vi "Publish Trace.vi"(8 "error in (no error)":errorcluster, 10 "Trace":refnum<class "Trace.lvclass">, 11 "Trace Controller in":refnum<class "Trace Controller.lvclass">) -> (0 "error out":errorcluster, 3 "Trace Controller out":refnum<class "Trace Controller.lvclass">)   [LabVIEW 2014, in "Robot Actor Framework.lvlib" / "Trace.lvlib" / "Trace Controller.lvclass"]
uses:
  Trace Controller.lvclass
  Trace Class/Trace.lvclass
  Trace Controller.lvclass/Trace Controller.ctl
  Trace Listener Messages/Published Trace Msg/Published Trace Msg.lvclass/Published Trace Msg.ctl
  <vilib>/ActorFramework/Message Enqueuer/Message Enqueuer.lvclass/Message Enqueuer.ctl
  <vilib>/ActorFramework/Message Enqueuer/Enqueue.vi
  <vilib>/ActorFramework/Message Priority Queue/Priority Enqueue.vi
  Trace Listener Messages/Published Trace Msg/Published Trace Msg.lvclass
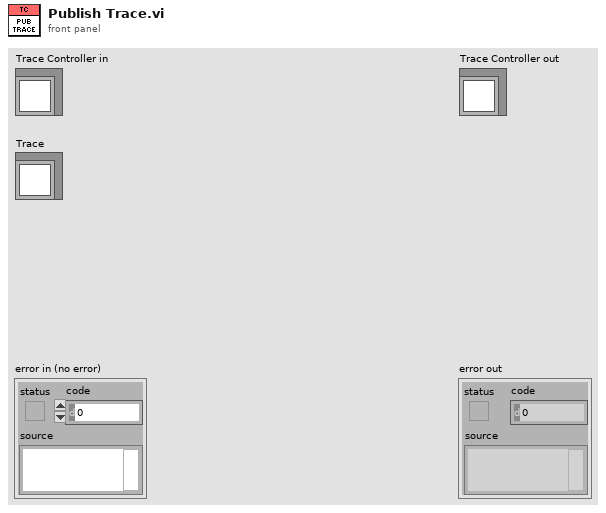
[diagram p1: front panel]
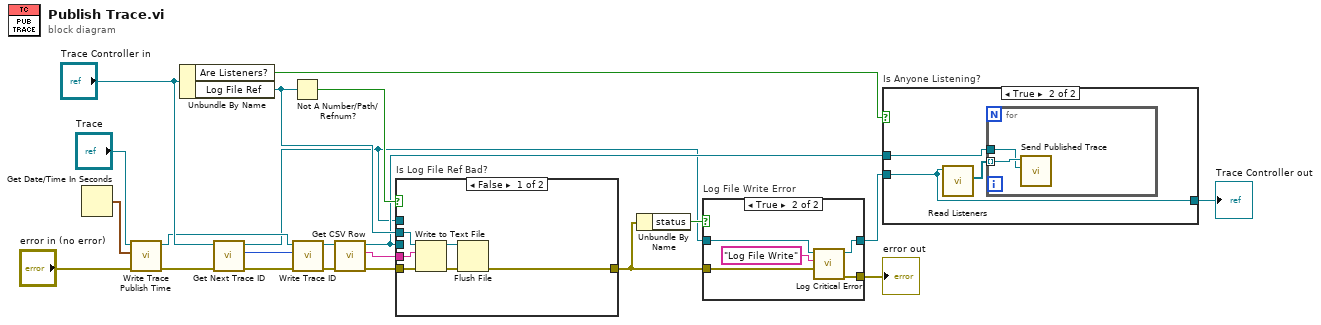
[diagram p0: block diagram]
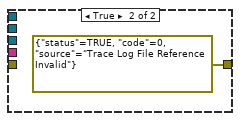
[diagram p2: hidden frame]
diagram:
  n1 = Get Date/Time In Seconds() -> (seconds since 1Jan1904=w19:timestamp)
  n2 = call-dynamic "Write Trace Publish Time.vi"("error in (no error)"="error in (no error)", "Trace Time"=w19, "Trace in"="Trace") -> ("error out"=w3:errorcluster, "Trace out"=w9:refnum<class "Trace.lvclass">)  [unwired: 7 in]
  n3 = Unbundle By Name("Trace Controller in") -> ("Are Listeners?"=w21:bool, "Log File Ref"=w12:refnum<file>)
  n4 = call-dynamic "Get Next Trace ID.vi"("error in (no error)"=w3, "Trace Controller in"="Trace Controller in") -> ("error out"=w2:errorcluster, "Next Trace ID"=w7:u64, "Trace Controller out"=w5:refnum<class "Trace Controller.lvclass">)  [unwired: 7 in]
  n5 = Not A Number/Path/Refnum?(number/path/refnum=w12) -> (NaN/Path/Refnum?=w11:bool)
  n6 = call-dynamic "Write Trace ID.vi"("error in (no error)"=w2, "Trace ID"=w7, "Trace in"=w9) -> ("error out"=w1:errorcluster, "Trace out"=w8:refnum<class "Trace.lvclass">)  [unwired: 7 in]
  n7 = call-dynamic "Get CSV Row.vi"("error in (no error)"=w1, "Trace in"=w8) -> ("error out"=w17:errorcluster, "CSV Row"=w18:string, "Trace out"=w6:refnum<class "Trace.lvclass">)  [unwired: 7 in]
  n8 = case "Is Log File Ref Bad?" shown="False" w11 {
    tunnel: w18 -> [w28 _]
    tunnel: w17 -> [w27 _]
    tunnel: [w25 errorcluster {"status"=TRUE, "code"=0, "source"="Trace Log File Reference Invalid"} ("error out")] -> w15
    tunnel: w12 -> [w26 _]
    tunnel: w6 -> [_ _]
    tunnel: w5 -> [_ _]
    frame False {
      n9 = Write to Text File(file (use dialog)=w26, text=w28, error in=w27) -> (refnum out=w24:refnum<file>, error out=w23:errorcluster)  [unwired: 1 in, 1 out]
      n10 = Flush File(refnum=w24, error in=w23) -> (error out=w25:errorcluster)  [unwired: 1 out]
    }
    frame True {
    }
  }
  n11 = Unbundle By Name(w15) -> ("status"=w16:bool)
  n12 = case "Log File Write Error" shown="True" w16 {
    tunnel: w5 -> [w31 w36]
    tunnel: w15 -> [w30 w34]
    tunnel: [w31 w33] -> w14
    tunnel: [w30 w32] -> w13
    frame False {
    }
    frame True {
      n13 = call-dynamic "Log Critical Error.vi"("Critical Error"=w34, "Critical Error Event"="Log File Write", "Trace Controller in"=w36) -> ("error out"=w32:errorcluster, "Trace Controller out"=w33:refnum<class "Trace Controller.lvclass">)  [unwired: 7 in]
    }
  }
  "error out" <- w13
  n14 = case "Is Anyone Listening?" shown="True" w21 {
    tunnel: w6 -> [_ w38]
    tunnel: w14 -> [w37 w39]
    tunnel: [w37 w39] -> w22
    frame False {
      # "If No One is Listening\nTo Traces, Do not Process\n To avoid Consuming\nResources"
    }
    frame True {
      n15 = call-dynamic "Read Listeners.vi"("Trace Controller in"=w39) -> ("Listeners"=w40:refnum<class "Message Enqueuer.lvclass">[])  [unwired: 8 in, 2 out]
      n16 = for {
        tunnel: w40 -> [w42] mode=indexing
        tunnel: w38 -> [w41]
        n17 = call "Send Published Trace.vi"("Trace"=w41, "Message Enqueuer"=w42) -> ()  [unwired: 8 in, 2 out]
      }
    }
  }
  "Trace Controller out" <- w22
